vi "top VI.vi"() -> ()   [LabVIEW 2014]
panel:
  in  "difficulty":i32(knob) scale=1.0..3.0
  in  "End Game":bool
  out "Game Array":picture[][](array[picture])
  # "Jiugongge picture puzzle"
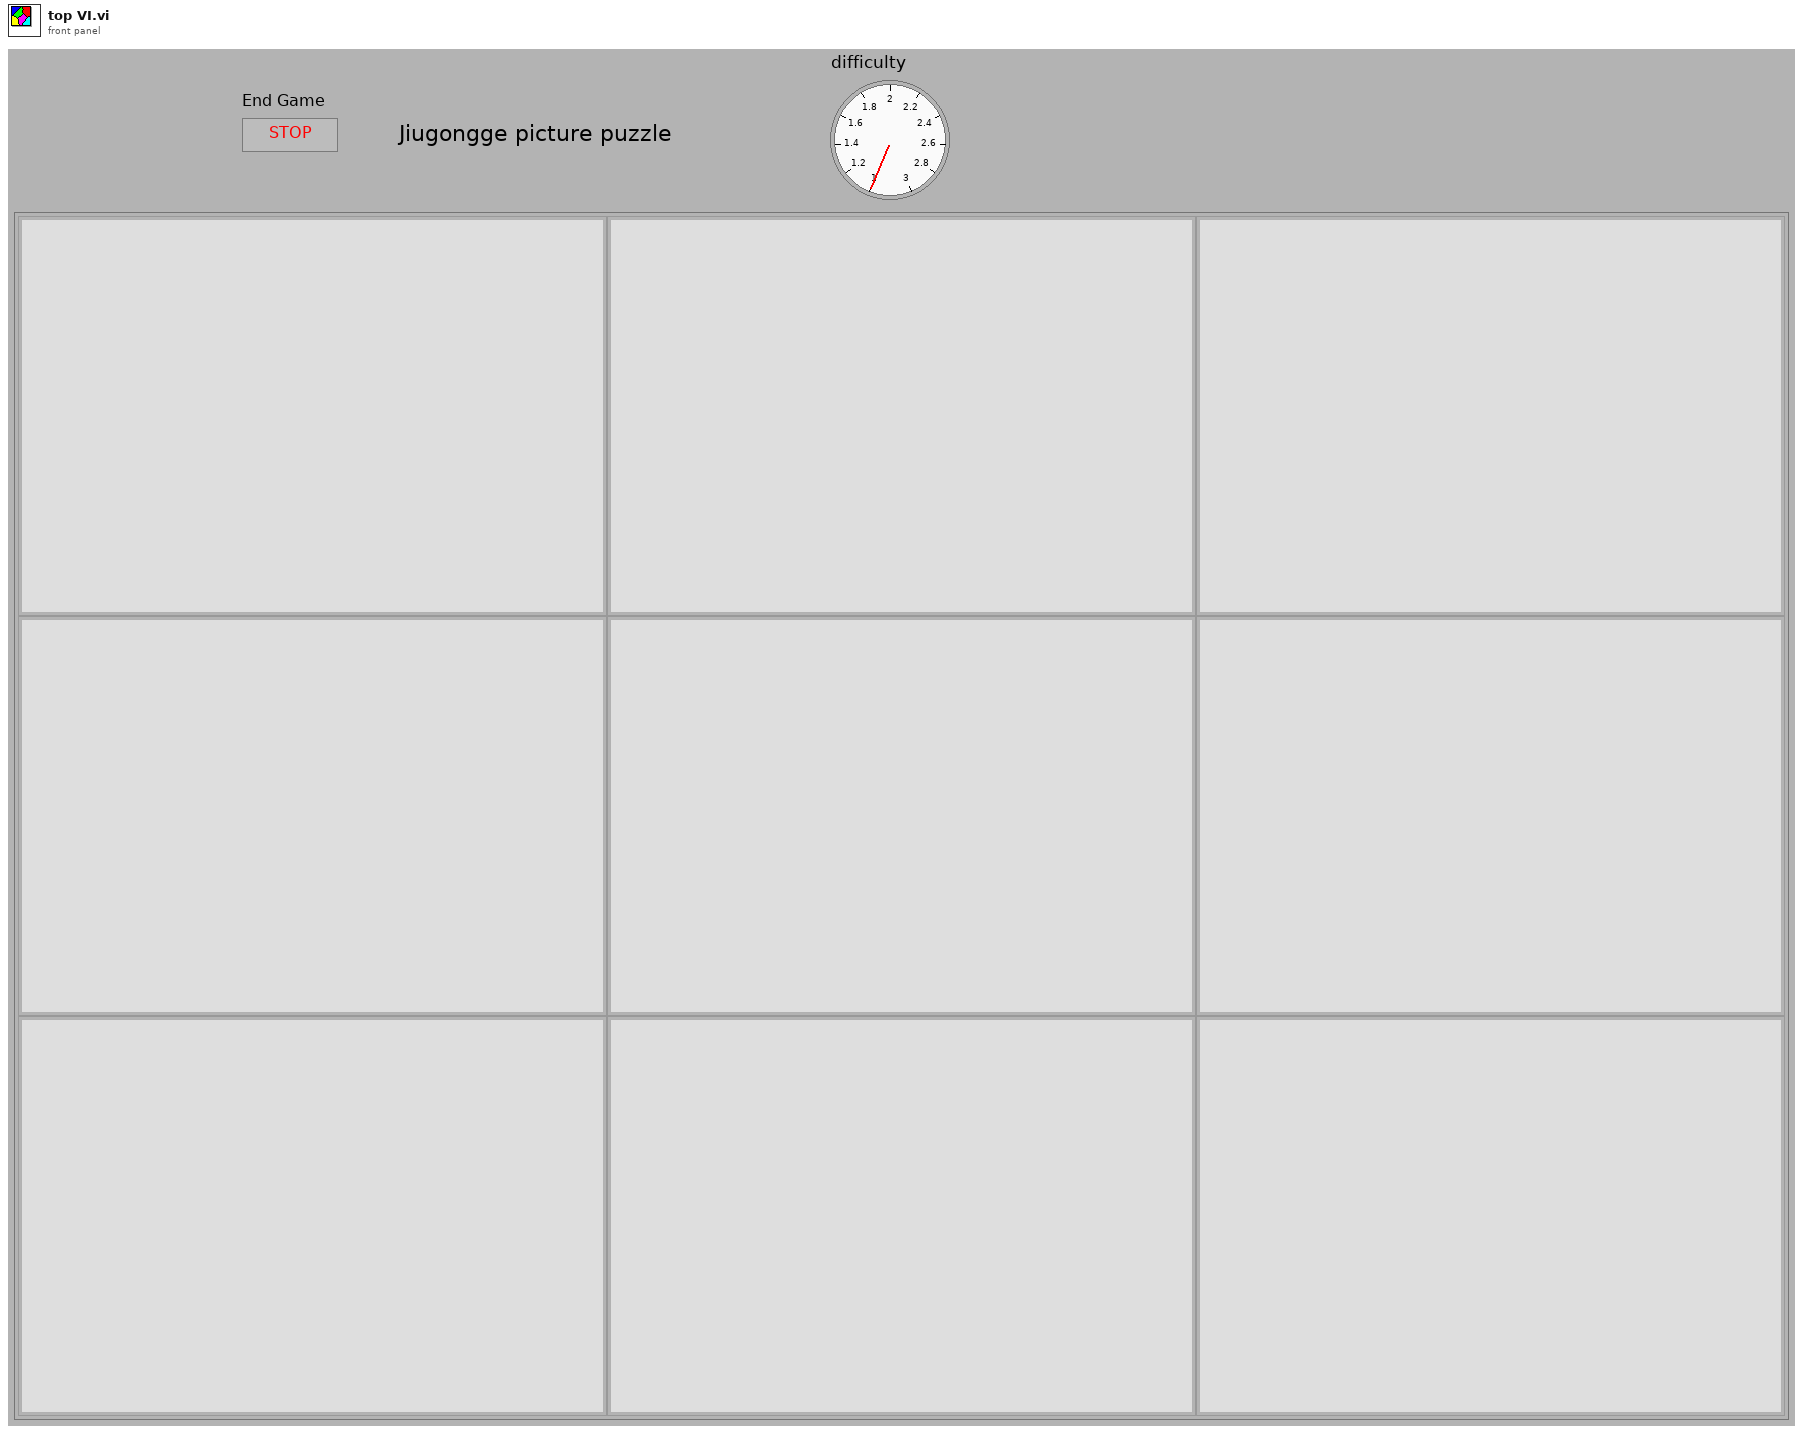
[diagram p1: front panel]
types:
  T1 = typedef "imagedata.ctl" = cluster{"image type":i32, "image depth":i32, "image":u8[], "mask":u8[], "colors":u32[], "Rectangle":cluster{"left":i16, "top":i16, "right":i16, "bottom":i16}}
  T2 = cluster{"Numeric Control":i32, "Numeric Control":i32}
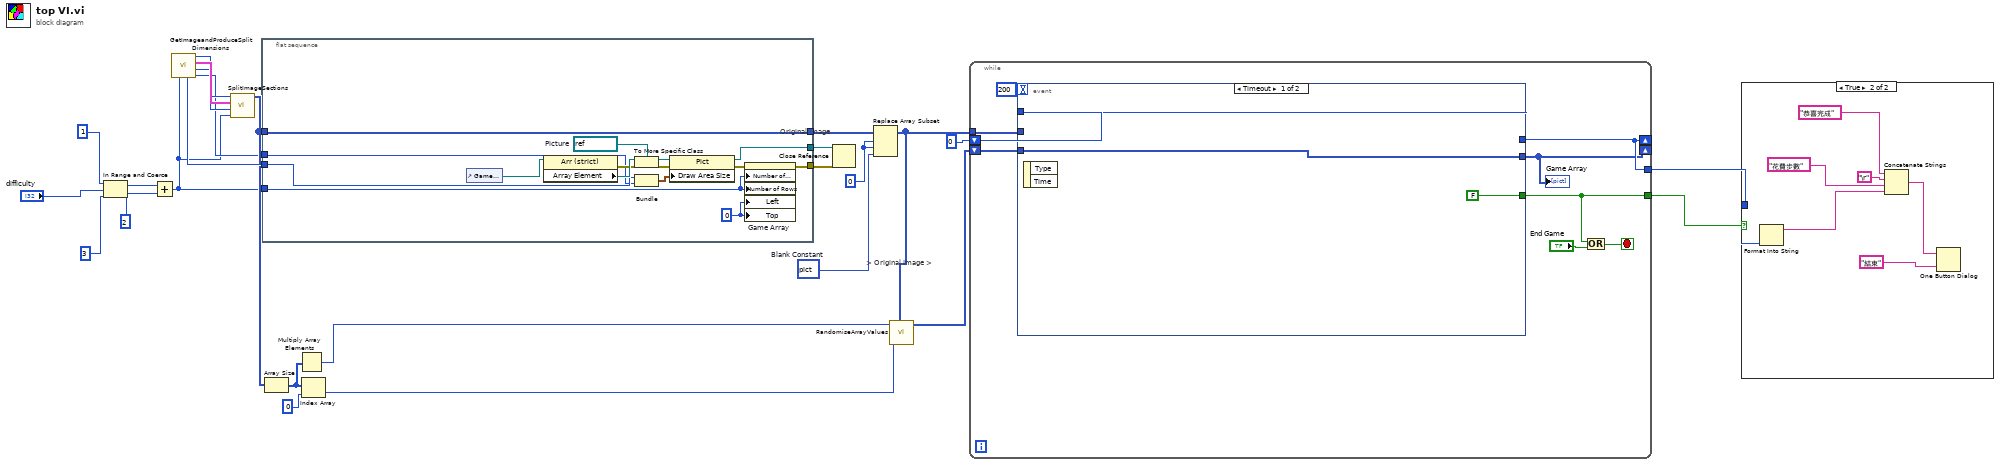
[diagram p0: block diagram]
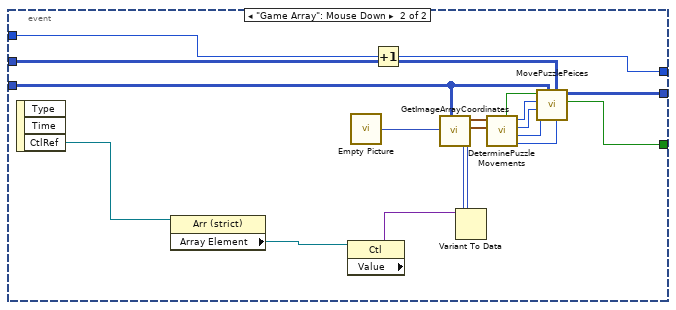
[diagram p3: hidden frame]
diagram:
  w15 = 0 ("index (row)")
  w16 = picture data[5B]  # Blank Constant
  # "Original Image"
  # "> Original Image >"
  n1 = In Range and Coerce(upper limit=1, x="difficulty", lower limit=3) -> (coerced(x)=w7:i32)  [unwired: 1 out]
  n2 = Add(x=w7, y=2) -> (x+y=w2:i32)
  n3 = call "GetImageandProduceSplitDimensions.vi"("length"=w2) -> ("size X"=w4:i32, "Y length"=w25:i32, "selected image"=w26:T1, "X length"=w24:i32, "size Y"=w20:i32)  [unwired: 6 in]
  n4 = call "SplitImageSections.vi"("array lenght (1D)"=w2, "y length"=w25, "selected image"=w26, "x length"=w24) -> ("chopped image array"=w8:picture[][])  [unwired: 7 in]
  n5 = flat-sequence {
    tunnel: w8 -> [w35]
    tunnel: [w35] -> w17
    tunnel: w20 -> [w34]
    tunnel: w4 -> [w28]
    tunnel: [w31] -> w18
    tunnel: [w33] -> w19
    tunnel: w2 -> [w30]
    frame #0 {
      w29 = 0 ("Position:Left")
      w38 = refnum<vi> refnum  # Picture
      n6 = control-ref of="Game Array"() -> (w41:refnum<vi>)
      n7 = property class="Arr (strict)"(reference=w41) -> (error out=w39:errorcluster, "Array Element"=w40:refnum<vi>)  [unwired: 1 in, 1 out]
      n8 = To More Specific Class(target class=w38, reference=w40, error in=w39) -> (specific class reference=w37:refnum<vi>, error out=w36:errorcluster)
      n9 = Bundle("size Y"=w34, "size X"=w28) -> (w27:cluster{"size Y":i32, "size X":i32})  [unwired: 1 in]
      n10 = property class="Pict"(reference=w37, error in=w36, "Draw Area Size"=w27) -> (reference out=w33:refnum<vi>, error out=w32:errorcluster)
      n11 = property on="Game Array" class="Arr (strict)"(error in=w32, "Number of Columns"=w30, "Number of Rows"=w30, "Left"=w29, "Top"=w29) -> (error out=w31:errorcluster)  [unwired: 1 in, 1 out]
    }
  }
  n12 = Array Size(array=w8) -> (size(s)=w22:i32[])
  n13 = Multiply Array Elements(1:w22) -> (0:w21:i32)
  n14 = Index Array(array=w22, index=0) -> (element=w10:i32)
  n15 = Close Reference(reference=w19, error in (no error)=w18) -> ()  [unwired: 1 out]
  n16 = Replace Array Subset(array=w17, new element=w16, index (row)=w15, index (col)=w15) -> (w3:picture[][])
  n17 = call "RandomiseArrayValues.vi"("original image"=w3, "maximumarray width/height"=w10, "total array elements"=w21) -> ("randomisedarray"=w14:picture[][])  [unwired: 8 in]
  n18 = while {
    shift-right: [w42] -> _
    shift-left: w14 -> [w49]
    tunnel: w3 -> [w48]
    tunnel: [w43] -> w1
    tunnel: [w45] -> w13
    shift-right: [w45] -> _
    shift-left: 0 -> [w46]
    stop <- w47 stop-if-true
    n19 = event shown="[0] Timeout" {
      selector: _ -> [_ _]
      dyn-events: _ -> [_ _]
      timeout: 200 -> [_ _]
      tunnel: w49 -> [w53 w58]
      tunnel: [w53 w64] -> w42
      tunnel: w48 -> [_ w59]
      tunnel: [FALSE w63] -> w43
      tunnel: w46 -> [w51 w62]
      tunnel: [w51 w61] -> w45
      event Timeout {
        n20 = event-data() -> ()  [unwired: 1 in, 2 out]
      }
      event "Game Array": Mouse Down {
        n21 = event-data() -> ("CtlRef"=w71:refnum<vi>)  [unwired: 1 in, 2 out]
        n22 = property class="Arr (strict)"(reference=w71) -> ("Array Element"=w70:refnum<vi>)  [unwired: 1 in, 2 out]
        n23 = property class="Ctl"(reference=w70) -> ("Value"=w69:variant)  [unwired: 1 in, 2 out]
        n24 = call "Empty Picture"() -> ("empty picture"=w68:picture)
        n25 = Increment(x=w62) -> (x+1=w61:i32)
        n26 = Variant To Data(type=w68, Variant=w69) -> (data=w60:picture)  [unwired: 1 in, 1 out]
        n27 = call "GetImageArrayCoordinates.vi"("current array"=w58, "image select"=w60) -> ("white Location out"=w66:T2, "peice Location out"=w67:T2)  [unwired: 8 in]
        n28 = call "DeterminePuzzleMovements.vi"(10:"location in"=w66, 11:"location in"=w67) -> ("upper white row position"=w55:i32, "current peice column"=w54:i32, "current peice row"=w65:i32, "lower white column position"=w56:i32, "allow [eice movement"=w57:bool)  [unwired: 5 in]
        n29 = call "MovePuzzlePeices.vi"("upper white row"=w55, "solve"=w59, "current state"=w58, "currentselected peice column"=w54, "current selected peice row"=w65, "lower white coordinate"=w56, "allow peice movement"=w57) -> ("puzzle finished"=w63:bool, "updated image array"=w64:picture[][])  [unwired: 3 in]
      }
    }
    "Game Array" <- w42
    n30 = Or(x=w43, y="End Game") -> (x .or. y?=w47:bool)
  }
  n31 = case shown="True" w1 {
    tunnel: w13 -> [_ w76]
    frame False {
    }
    frame True {
      n32 = Format Into String(w76) -> (resulting string=w75:string)  [unwired: 3 in, 1 out]
      n33 = Concatenate Strings("恭喜完成" ("message"), "\r", "花費步數" ("string"), w75) -> (w77:string)
      n34 = One Button Dialog(message=w77, button name ("OK")="結束") -> ()  [unwired: 1 out]
    }
  }
